vi "Construct_Log_File_Path.vi"(8 "error in (no error)":errorcluster, 10 "filename without extension":string, 11 "build":refnum<class "AB_Build.lvclass">) -> (0 "error out":errorcluster, 3 "appended path":path)   [LabVIEW 2020, in "AB_Deployment.lvlib"]
uses:
  <vilib>/AppBuilder/AB_Classes/Deployment/AB_Deployment.lvlib
  <vilib>/AppBuilder/AB_Classes/Build/AB_Build.lvclass
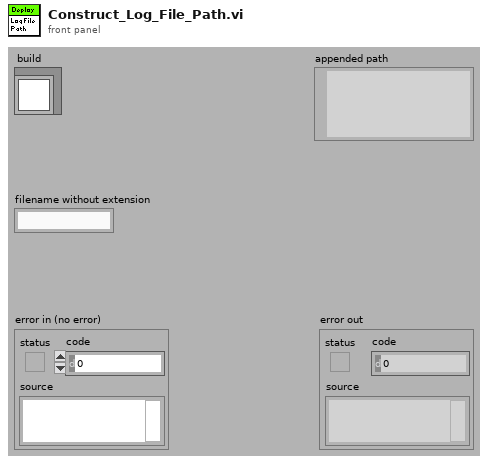
[diagram p1: front panel]
types:
  T1 = typedef "AB_Build.ctl" = cluster{"buildSpecName":string, "buildSpecDescription":string, "destinations":refnum<class "AB_Destination.lvclass">[], "exclusionOption":T2, "defaultLanguage":string, "supportedLanguages":string[], "excludedDirectories":path[], "buildContext":refnum<vi>, "buildObject":T3, "preview":bool, "programatic":bool, "progressBarEvents":T4, "userLog_Path":path, "preActionID":string, "preAction_Path":path, "postActionID":string, "postAction_Path":path, "eng_checkForBrokenVIs?":bool, "eng_verboseLinkerErrors?":bool, "localDest_Path":path, "targetDest_Path":path, "removeVIObject":u16, "cache":refnum<class "PreviewCache.lvclass">, "use cache":bool, "previewCache_ID":string, "buildCache_ID":string, "eng_TempLocalDest_Path":path, "eng_collectDependencies?":bool, "versionInfo":cluster{"buildVersion":cluster{"major":u16, "minor":u16, "patch":u16, "build":u16}, "autoIncrement":bool}, "eng_enableVIChecksums":bool}
  T2 = typedef "AB_Exclusion_Option.ctl" = cluster{"typedefs":bool, "polymorphicVIs":bool, "unusedLibraryItems":bool, "modifyLibraryFile":bool, "edit-timeDependencies":bool, "inlineVIs":bool, "dependent PPLs":bool, "dependent DLLs":bool}
  T3 = typedef "ItemRef.ctl" = u64
  T4 = typedef "provcom_ProgressBar_Events.ctl" = cluster{"newJob":refnum<user-event>, "newItem":refnum<user-event>, "errorMsg":T5, "cancel":refnum<user-event>}
  T5 = typedef "mxLvBuildError.ctl" = refnum<user-event>
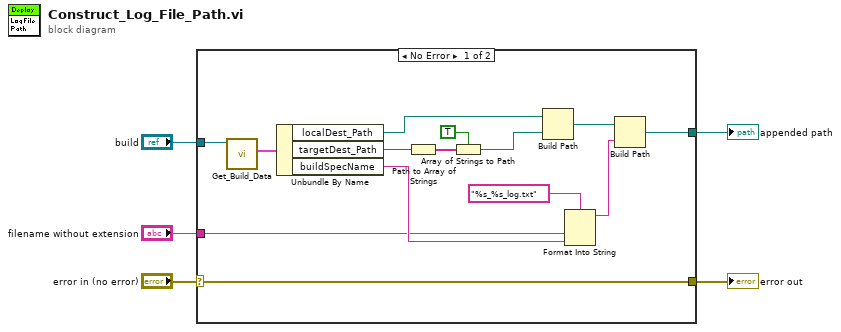
[diagram p0: block diagram]
diagram:
  n1 = case shown="No Error" "error in (no error)" {
    selector: "error in (no error)" -> [w12 w20]
    tunnel: "build" -> [w15 _]
    tunnel: [w14 _] -> w4
    tunnel: "filename without extension" -> [w13 _]
    tunnel: [w12 w20] -> w1
    frame No Error {
      n2 = call <vilib>:"Get_Build_Data.vi"("Class in"=w15) -> ("data"=w16:T1)  [unwired: 8 in, 2 out]
      n3 = Unbundle By Name(w16) -> ("localDest_Path"=w8:path, "targetDest_Path"=w7:path, "buildSpecName"=w19:string)
      n4 = Path to Array of Strings(0:w7) -> (2:w11:string[])  [unwired: 1 out]
      n5 = Array of Strings to Path(0:w11, 1:TRUE ("relative")) -> (2:w9:path)
      n6 = Build Path(base path=w8, name or relative path=w9) -> (appended path=w6:path)
      n7 = Format Into String(format string="%s_%s_log.txt", w13, w19) -> (resulting string=w18:string)  [unwired: 2 in, 1 out]
      n8 = Build Path(base path=w6, name or relative path=w18) -> (appended path=w14:path)
    }
    frame Error {
    }
  }
  "appended path" <- w4
  "error out" <- w1
